vi "Write_parameter.vi"(8 "error in (no error)":errorcluster caption="entrée d'erreur (pas d'erreur)", 10 "Parameter":string, 11 "Class Instrument Process en entrée":refnum<class "Class Instrument Process.lvclass">) -> (0 "error out":errorcluster caption="sortie d'erreur", 3 "Class Instrument Process en sortie":refnum<class "Class Instrument Process.lvclass">)   [LabVIEW 2020, in "Library Instrument & Equipement.lvlib" / "Library Instruments.lvlib" / "Class Instrument Process.lvclass"]
uses:
  Class Instrument Process.lvclass
  Commun VI/TypeDef/Commande Process/Parameter Process.ctl
  Process/Process (Default)/Process (Default).lvclass
  JSON API/JSON Value/Set from JSON string.vi
  Instrument (Default)/Class Instrument (Default).lvclass
  JSON API/JSON Value/JSON Value.lvclass
  Class Instrument Process.lvclass/Class Instrument Process.ctl
  JSON API/Variant JSON/Variant JSON.lvlib
  JSON API/Get Polymorphic/JSON GetSet.lvlib
  Commun VI/Library Commun.lvlib
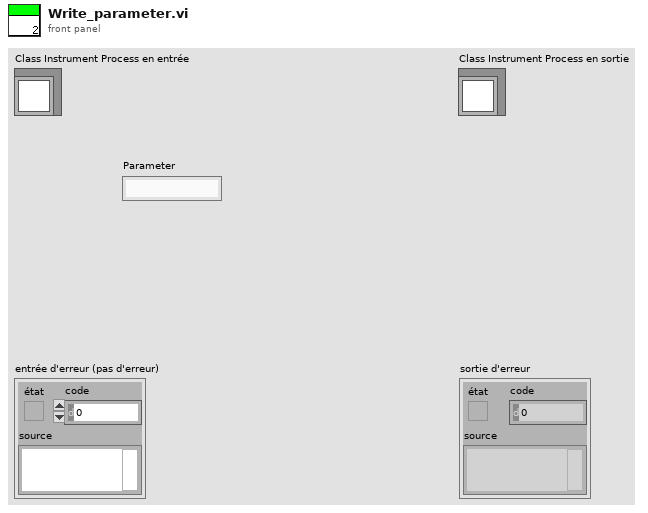
[diagram p1: front panel]
types:
  T1 = typedef "Library Commun.lvlib/Parameter Process.ctl" = cluster{"FileName":string, "Arguments":string, "Working Directory":string, "Class Process":refnum<class "Process (Default).lvclass">}
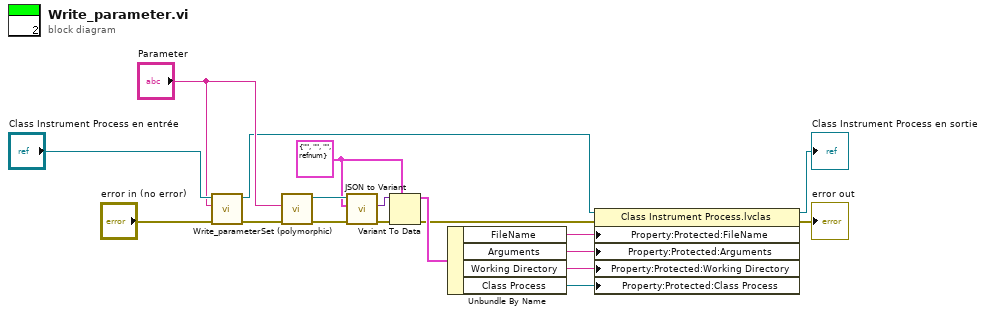
[diagram p0: block diagram]
diagram:
  w10 = T1 {"FileName"="", "Arguments"="", "Working Directory"="", "Class Process"=refnum} ("Parameter")
  n1 = call-parent "Write_parameter.vi"("error in (no error)"="error in (no error)", "Parameter"="Parameter", "Class Instrument (Default) en entrée"="Class Instrument Process en entrée") -> ("error out"=w12:errorcluster, "Class Instrument (Default) en sortie"=w8:refnum<class "Class Instrument Process.lvclass">)  [unwired: 7 in]
  n2 = call-poly "Set (polymorphic).vi"("error in (no error)"=w12, "JSON stream"="Parameter") -> ("error out"=w14:errorcluster, "JSON Value out"=w16:refnum<class "JSON Value.lvclass">)  [unwired: 7 in, 1 out]
  n3 = call "JSON to Variant.vi"("error in (no error)"=w14, "Variant (Data Type)"=w10, "JSON Value"=w16) -> ("error out"=w15:errorcluster, "Variant out"=w13:variant)  [unwired: 7 in]
  n4 = Variant To Data(error in=w15, type=w10, Variant=w13) -> (data=w9:T1, error out=w6:errorcluster)
  n5 = Unbundle By Name(w9) -> ("FileName"=w5:string, "Arguments"=w4:string, "Working Directory"=w3:string, "Class Process"=w2:refnum<class "Process (Default).lvclass">)
  n6 = property class="Class Instrument Process.lvclas"(reference=w8, error in=w6, "Property:Protected:FileName"=w5, "Property:Protected:Arguments"=w4, "Property:Protected:Working Directory"=w3, "Property:Protected:Class Process"=w2) -> (reference out=→"Class Instrument Process en sortie":refnum<class "Class Instrument Process.lvclass">, error out=→"error out":errorcluster)
